vi "Strain_Gauge_Control.vi"() -> ()   [LabVIEW 2015]
panel:
  in  "Null":bool
  in  "measure":bool
  out "Date/time":string
  in  "Names:":string
  out "e_meas vs. P":cluster{dbl[], dbl[]}(graph)
  out "% Error":dbl
  in  "Material":string
  out "e_meas (Unloaded)":dbl format="%e"
  out "stdv unloaded":dbl format="%e"
  out "e_meas (Loaded)":dbl format="%e"
  out "stdv loaded":dbl format="%e"
  in  "stop":bool
  out "AI.Bridge.InitialVoltage [mV]":dbl format="%_6g"
  in  "Strain physical channels":tag
  out "e_theo":dbl
  in  "Young's Modulus, E [GPa]":dbl
  in  "Thickness, t [mm]":dbl
  in  "Width, w [mm]":dbl
  in  "Load Applied, P [kg]":dbl
  in  "Distance from end to strain gauge, l [mm]":dbl
  in  "Length, L [mm]":dbl
  # "5. Add Load to Beam"
  # "1. Select the Strain Gauge Channel"
  # "3. Run the Program (CTRL+R)"
  # "For Each Load, Enter Value"
  # "And Record Names"
  # "4. With NO LOAD,   Offset Null"
  # "Take Measurement"
  # "2. Enter Material Properties"
  # "Repeat for All Desired Loads"
  # "Current Load Data"
  # "6. To Finish, Press ABORT (CTRL+.)"
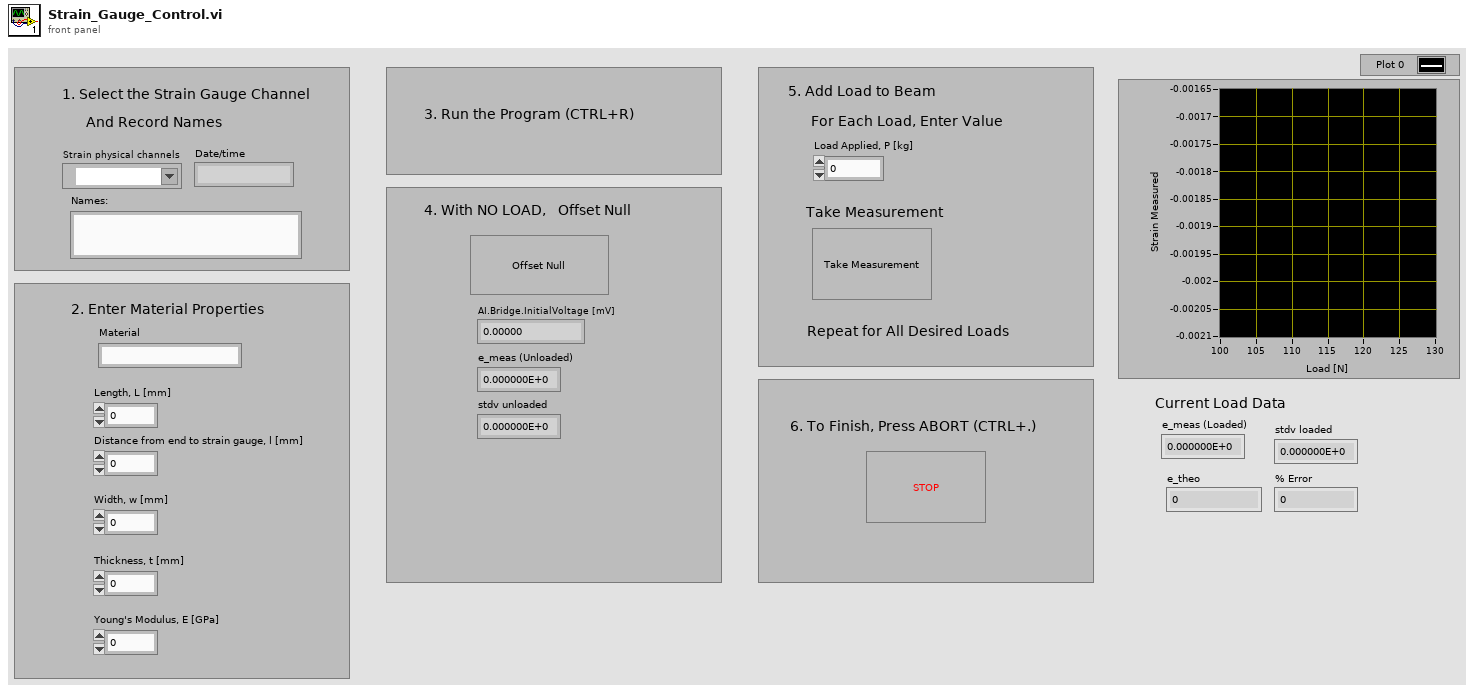
[diagram p1: front panel]
types:
  T1 = enum16{"open", "replace", "create", "open or create", "replace or create", "replace or create with confirmation"}
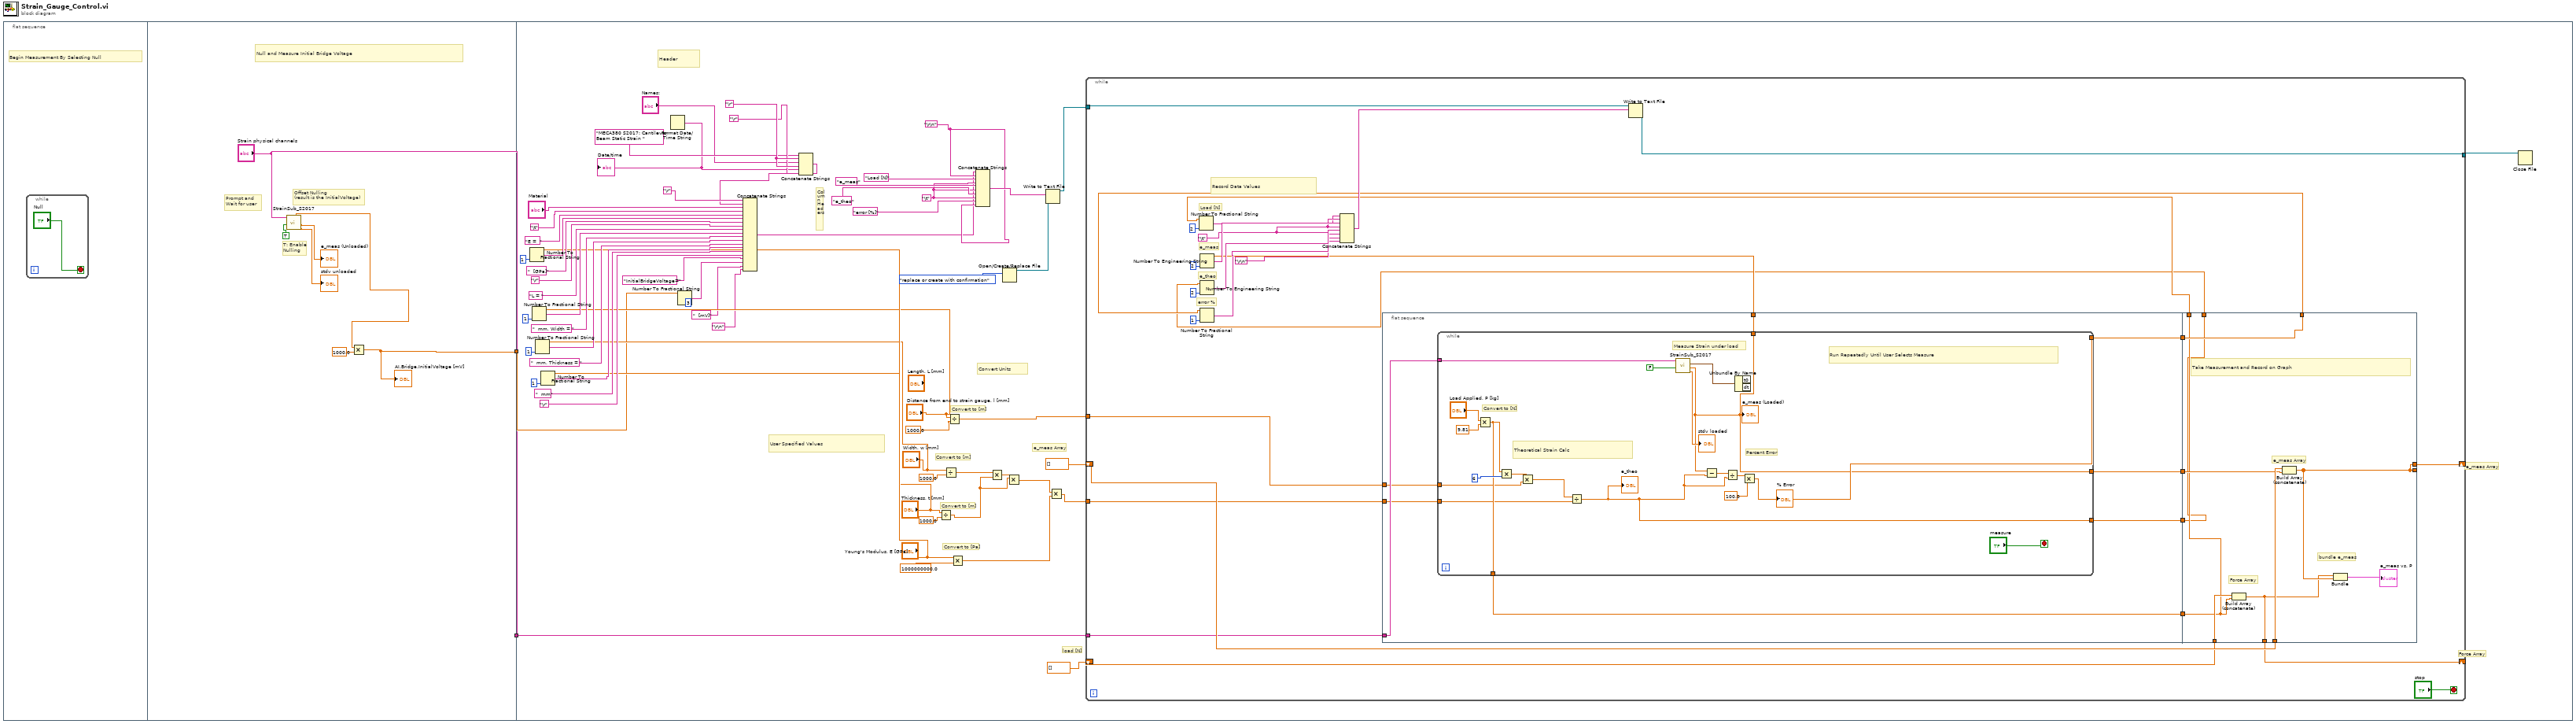
[diagram p0: block diagram]
diagram:
  n1 = flat-sequence {
    tunnel: ["Strain physical channels"] -> w2
    tunnel: [w7] -> w1
    tunnel: w2 -> [w19]
    tunnel: w1 -> [w18]
    frame #0 {
      # "Begin Measurement By Selecting Null"
      n2 = while {
        stop <- "Null" stop-if-true
      }
    }
    frame #1 {
      # "Offset Nulling\n(result is the InitialVoltage)"
      # "T: Enable\nNulling"
      # "Null and Measure Initial Bridge Voltage"
      # "Prompt and\nWait for user"
      n3 = call "StrainSub_S2017.vi"("physical channels"="Strain physical channels", "Offset Null?"=TRUE ("Do Offset Null?")) -> ("AI.Bridge.InitialVoltage"=w9:dbl, "mean"=→"e_meas (Unloaded)":dbl, "standard deviation"=→"stdv unloaded":dbl)  [unwired: 2 in, 2 out]
      n4 = Multiply(x=w9, y=1000.0) -> (x*y=w7:dbl)
      "AI.Bridge.InitialVoltage [mV]" <- w7
    }
    frame #2 {
      w68 = "\r"
      w57 = "\t"
      w56 = "\r\n"
      # "User Specified Values"
      # "Convert Units"
      # "load [N]"
      # "Convert to [m]"
      # "Convert to [Pa]"
      # "Convert to [m]"
      # "Convert to [m]"
      # "Header"
      # "Column Headers"
      # "e_meas Array"
      # "e_meas Array"
      # "Force Array"
      n5 = Number To Fractional String(number="Young's Modulus, E [GPa]", precision (6)=i16 1) -> (F-format string=w42:string)  [unwired: 2 in]
      n6 = Number To Fractional String(number="Distance from end to strain gauge, l [mm]", precision (6)=i16 1) -> (F-format string=w37:string)  [unwired: 2 in]
      n7 = Number To Fractional String(number="Width, w [mm]", precision (6)=i16 1) -> (F-format string=w34:string)  [unwired: 2 in]
      n8 = Number To Fractional String(number="Thickness, t [mm]", precision (6)=i16 1) -> (F-format string=w31:string)  [unwired: 2 in]
      n9 = Format Date/Time String() -> (date/time string=w64:string)  [unwired: 3 in]
      "Date/time" <- w64
      n10 = Number To Fractional String(number=w18, precision (6)=i16 3) -> (F-format string=w20:string)  [unwired: 2 in]
      n11 = Concatenate Strings("MECA380 S2017: Cantilever Beam Static Strain ", w68, "Names:", w68, w64, "\r") -> (w28:string)
      n12 = Concatenate Strings("\r", w28, "Material", "\t", "E =  ", w42, "  [GPa]", "\r", "L = ", w37, "  mm, Width = ", w34, "  mm, Thickness = ", w31, "  mm", "\r", "InitialBridgeVoltage=", w20, "  [mV]", "\r\n") -> (w27:string)
      n13 = Divide(x="Thickness, t [mm]", y=1000.0) -> (x/y=w48:dbl)
      n14 = Divide(x="Width, w [mm]", y=1000.0) -> (x/y=w50:dbl)
      n15 = Divide(x="Distance from end to strain gauge, l [mm]", y=1000.0) -> (x/y=w14:dbl)
      n16 = Multiply(x="Young's Modulus, E [GPa]", y=1000000000.0) -> (x*y=w12:dbl)
      n17 = Concatenate Strings(w27, w56, "Load [N]", w57, "e_meas", w57, "e_theo", w57, "error [%]", w56) -> (w60:string)
      n18 = Multiply(x=w50, y=w48) -> (x*y=w49:dbl)
      n19 = Open/Create/Replace File(operation (0:open)=T1."replace or create with confirmation" ("Output:")) -> (refnum out=w62:refnum<file>)  [unwired: 5 in, 2 out]
      n20 = Multiply(x=w48, y=w49) -> (x*y=w13:dbl)
      n21 = Write to Text File(file (use dialog)=w62, text=w60) -> (refnum out=w22:refnum<file>)  [unwired: 2 in, 2 out]
      n22 = Multiply(x=w13, y=w12) -> (x*y=w11:dbl)
      n23 = while {
        shift-right: [w72] -> _
        shift-left: dbl[] [] -> [w79]
        shift-right: [w81] -> _
        shift-left: dbl[] [] -> [w91]
        tunnel: [w89] -> w55
        tunnel: w22 -> [w88]
        tunnel: w19 -> [w87]
        tunnel: w14 -> [w76]
        tunnel: w11 -> [w75]
        stop <- "stop" stop-if-true
        w94 = "\t"
        # "Record Data Values"
        # "error %"
        # "e_theo"
        # "e_meas"
        # "Load [N]"
        n24 = Number To Fractional String(number=w77, precision (6)=i16 2) -> (F-format string=w86:string)  [unwired: 2 in]
        n25 = Number To Engineering String(2:i16 2 ("precision (6)"), 4:w82) -> (0:w98:string)  [unwired: 2 in]
        n26 = Number To Engineering String(2:i16 2 ("precision (6)"), 4:w74) -> (0:w96:string)  [unwired: 2 in]
        n27 = Number To Fractional String(number=w85, precision (6)=i16 1) -> (F-format string=w93:string)  [unwired: 2 in]
        n28 = Concatenate Strings(w86, w94, w98, w94, w96, w94, w93, "\r\n") -> (w90:string)
        n29 = flat-sequence {
          tunnel: w87 -> [w108]
          tunnel: [w107] -> w84
          tunnel: [w106] -> w83
          tunnel: [w105] -> w82
          tunnel: [w104] -> w78
          tunnel: w76 -> [w103]
          tunnel: w75 -> [w102]
          tunnel: [w101] -> w73
          tunnel: w91 -> [w136]
          tunnel: [w133] -> _
          tunnel: [w135] -> w85
          tunnel: w84 -> [w135]
          tunnel: w83 -> [w134]
          tunnel: [w133] -> w81
          tunnel: w79 -> [w132]
          tunnel: w78 -> [w130]
          tunnel: [w130] -> w77
          tunnel: [w129] -> w74
          tunnel: w73 -> [w129]
          tunnel: [w128] -> w72
          frame #0 {
            n30 = while {
              tunnel: w108 -> [w121]
              tunnel: [w120] -> w107
              tunnel: [w119] -> w106
              tunnel: [w119] -> w105
              tunnel: [w112] -> w104
              tunnel: w103 -> [w111]
              tunnel: w102 -> [w110]
              tunnel: [w109] -> w101
              stop <- "measure" stop-if-true
              # "Convert to [N]"
              # "Theoretical Strain Calc"
              # "Run Repeatedly Until User Selects Measure"
              # "Percent Error"
              # "Measure Strain under load"
              n31 = Multiply(x="Load Applied, P [kg]", y=9.81) -> (x*y=w112:dbl)
              n32 = Multiply(x=w112, y=6) -> (x*y=w115:dbl)
              n33 = Multiply(x=w115, y=w111) -> (x*y=w117:dbl)
              n34 = Divide(x=w117, y=w110) -> (x/y=w109:dbl)
              "e_theo" <- w109
              n35 = call "StrainSub_S2017.vi"("physical channels"=w121, "Offset Null?"=FALSE) -> ("Waveform Graph"=w123:waveform(dbl), "mean"=w119:dbl, "standard deviation"=→"stdv loaded":dbl)  [unwired: 2 in, 2 out]
              "e_meas (Loaded)" <- w119
              n36 = Subtract(x=w119, y=w109) -> (x-y=w126:dbl)
              n37 = Divide(x=w126, y=w109) -> (x/y=w125:dbl)
              n38 = Unbundle By Name(w123) -> ()  [unwired: 2 out]
              n39 = Multiply(x=w125, y=100.0) -> (x*y=w120:dbl)
              "% Error" <- w120
            }
          }
          frame #1 {
            # "Force Array"
            # "e_meas Array"
            # "Take Measurement and Record on Graph"
            # "bundle e_meas"
            n40 = Build Array (concatenate)(w132, w130) -> (w128:dbl[])
            n41 = Build Array (concatenate)(w136, w134) -> (w133:dbl[])
            n42 = Bundle(w128, w133) -> (→"e_meas vs. P":cluster{dbl[], dbl[]})  [unwired: 1 in]
          }
        }
        n43 = Write to Text File(file (use dialog)=w88, text=w90) -> (refnum out=w89:refnum<file>)  [unwired: 2 in, 2 out]
      }
      n44 = Close File(refnum=w55) -> ()  [unwired: 1 in, 2 out]
    }
  }
